vi "Nature_of_the_Person.vi"(0 "Application_Directory":path, 4 "Finish?":T1, 11 "Error_In":errorcluster) -> (15 "Error_Out":errorcluster)   [LabVIEW 2021]
doc: "This is a VI work as one of the front panel of the Game asking, the showing result about them."
uses:
  Controls/State.ctl
  Controls/Bool_Button.ctl
panel:
  out "NotP_Out":string
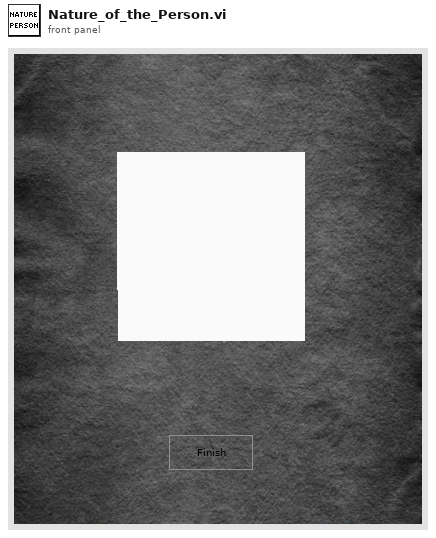
[diagram p1: front panel]
types:
  T1 = typedef "Bool_Button.ctl" = bool
  T2 = enum32{"Invalid", "Standard", "Closed", "Hidden", "Minimized", "Maximized"}
  T3 = typedef "State.ctl" = enum16{"Close", "Password_Popup", "Start_Popup", "Wizard_Msg", "Get_Name_DoB", "Lucky_Number", "Q-1", "Q-2", "Q-3", "Nature_of_the_Person"}
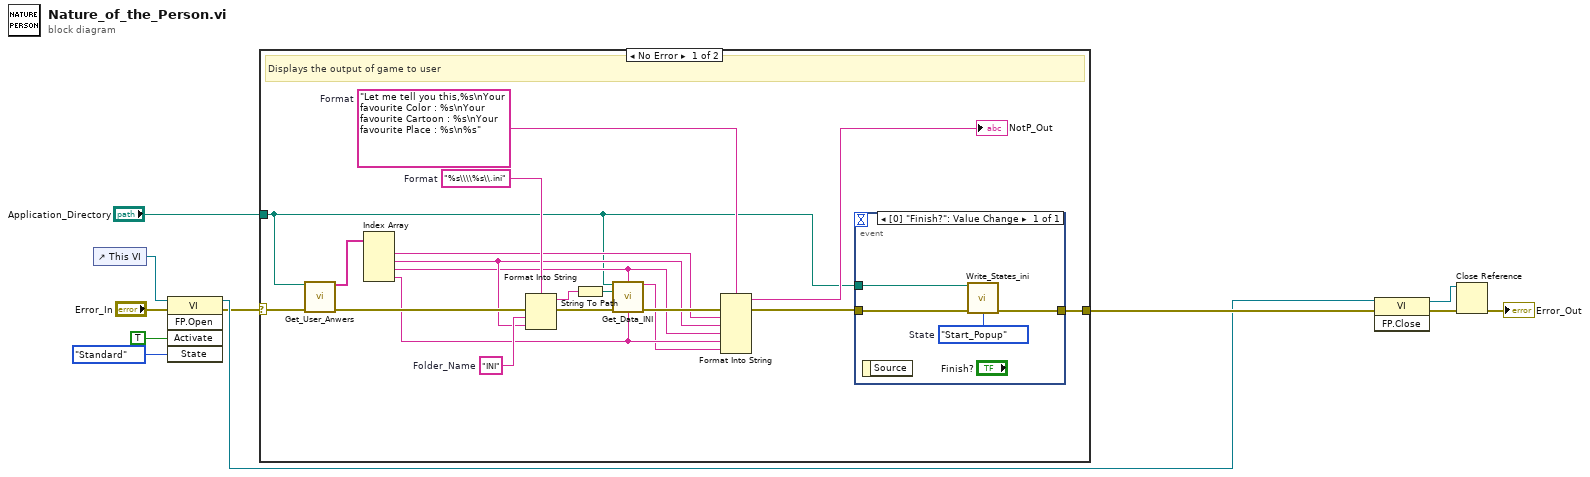
[diagram p0: block diagram]
diagram:
  n1 = control-ref of="This VI"() -> (w9:refnum<vi>)
  n2 = invoke class="VI" method="FP.Open"(reference=w9, error in="Error_In", "Activate"=TRUE ("Activate?"), "State"=T2."Standard") -> (reference out=w4:refnum<vi>, error out=w2:errorcluster)  [unwired: 1 in, 3 out]
  n3 = case shown="No Error" w2 {
    selector: w2 -> [w20 w35]
    tunnel: [w30 w35] -> w10
    tunnel: "Application_Directory" -> [w12 _]
    frame No Error {
      w21 = "INI"  # Folder_Name
      w22 = "%s\\\\%s\\.ini"  # Format
      w27 = "Let me tell you this,%s\nYour favourite Color : %s\nYour favourite Cartoon : %s\nYour favourite Place : %s\n%s"  # Format
      # "Displays the output of game to user"
      n4 = call "Get_User_Anwers.vi"("Application_Directory"=w12, "Error_In"=w20) -> ("User_Answer"=w29:string[], "Error_Out"=w19:errorcluster)  [unwired: 12 in]
      n5 = Index Array(array=w29) -> (element #1=w17:string, element #2=w16:string, element #3=w15:string, element #4=w14:string)  [unwired: 4 in]
      n6 = Format Into String(format string=w22, error in=w19, w21, w16) -> (resulting string=w24:string, error out=w23:errorcluster)  [unwired: 1 in]
      n7 = String To Path(string=w24) -> (path=w25:path)
      n8 = call "Get_Data_INI.vi"("Application_Directory"=w12, "Section"=w15, "File_Name"=w25, "Error_In"=w23, "Key"=w14) -> ("Data"=w13:string, "Error_Out"=w18:errorcluster)  [unwired: 9 in]
      n9 = Format Into String(format string=w27, error in=w18, w17, w16, w15, w14, w13) -> (resulting string=→"NotP_Out":string, error out=w28:errorcluster)  [unwired: 1 in]
      n10 = event shown="[0] \"Finish?\": Value Change" {
        selector: _ -> [_]
        dyn-events: _ -> [_]
        timeout: _ -> [_]
        tunnel: w28 -> [w34]
        tunnel: [w33] -> w30
        tunnel: w12 -> [w31]
        event Value Change {
          w32 = State."Start_Popup"  # State
          n11 = event-data() -> ()  [unwired: 1 in, 1 out]
          n12 = call "Write_States_ini.vi"("Application_Directory"=w31, "Error_In"=w34, "State"=w32) -> ("Error_Out"=w33:errorcluster)  [unwired: 12 in]
        }
      }
    }
    frame Error {
    }
  }
  n13 = invoke class="VI" method="FP.Close"(reference=w4, error in=w10) -> (reference out=w5:refnum<vi>, error out=w7:errorcluster)  [unwired: 1 in, 1 out]
  n14 = Close Reference(reference=w5, error in (no error)=w7) -> (error out=→"Error_Out":errorcluster)
